vi "DSF.Engine.Pool.ID.Return ID to Pool.vi"(8 "error in (no error)":errorcluster, 9 "timeout in ms (0)":i32 format="%d ms", 10 "id":i32, 11 "ID Pool in":refnum<class "DSF.Engine.Pool.ID.lvclass">) -> (0 "error out":errorcluster, 1 "timed out?":bool, 3 "ID Pool out":refnum<class "DSF.Engine.Pool.ID.lvclass">)   [LabVIEW 2017, in "DSF.Engine.lvlib" / "DSF.Engine.Pool.ID.lvclass"]
uses:
  DSF.Engine.Pool.ID.lvclass
  C:/Git/DSF/Source/Engine/Classes/Thread Pool/DSF.Engine.Pool.lvclass
  DSF.Engine.Pool.lvclass/DSF.Engine.Pool.ctl
  DSF.Engine.Pool.Get FIFO.vi
  DSF.Engine.Pool.lvclass
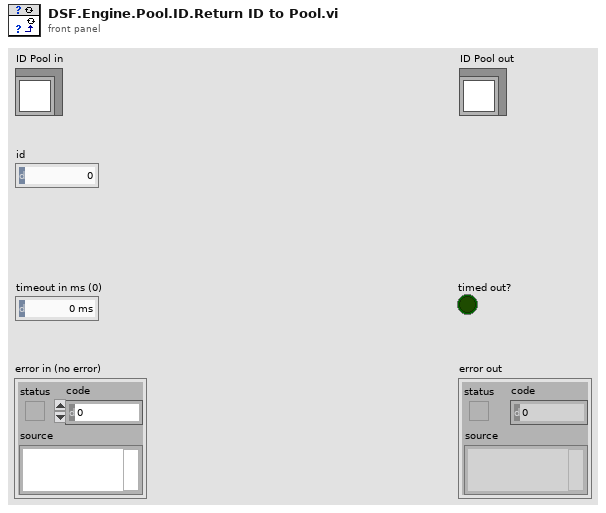
[diagram p1: front panel]
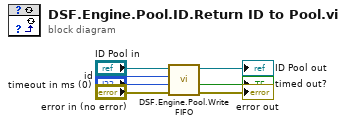
[diagram p0: block diagram]
diagram:
  n1 = call "DSF.Engine.Pool.Write FIFO.vi"("error in (no error)"="error in (no error)", "timeout in ms (0)"="timeout in ms (0)", "element"="id", "Pool in"="ID Pool in") -> ("error out"=→"error out":errorcluster, "timed out?"=→"timed out?":bool, "Pool out"=→"ID Pool out":refnum<class "DSF.Engine.Pool.ID.lvclass">)  [unwired: 5 in]
